vi "Get Cooler Status.vi"(8 "error in (no error)":errorcluster, 11 "CCDCamera in":refnum<class "CCDCamera.lvclass">) -> (0 "error out":errorcluster, 3 "CCDCamera out":refnum<class "CCDCamera.lvclass">)   [LabVIEW 2018, in "CCDCamera.lvclass"]
uses:
  CCDCamera.lvclass
  CCDCamera.lvclass/CCDCamera.ctl
  Cooler/Cooler.lvclass
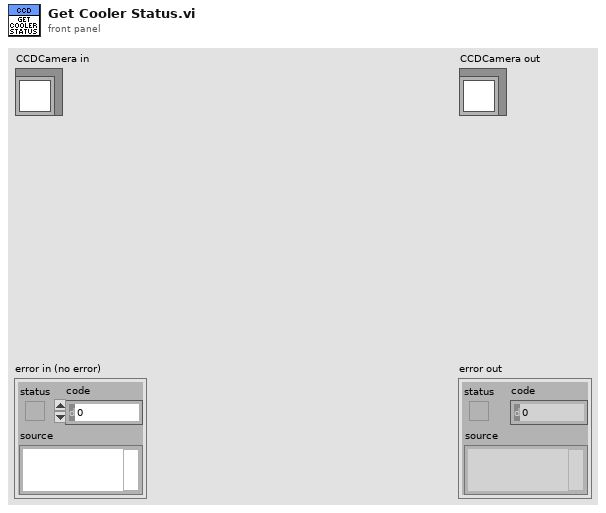
[diagram p1: front panel]
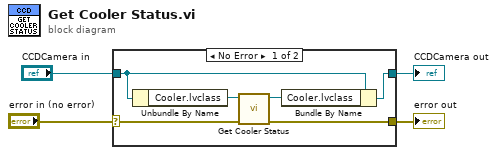
[diagram p0: block diagram]
diagram:
  n1 = case shown="No Error" "error in (no error)" {
    selector: "error in (no error)" -> [w5 w12]
    tunnel: [w6 w12] -> w3
    tunnel: [w8 w11] -> w1
    tunnel: "CCDCamera in" -> [w9 w11]
    frame No Error {
      n2 = Unbundle By Name(w9) -> ("Cooler.lvclass"=w10:refnum<class "Cooler.lvclass">)
      n3 = call "Get Cooler Status.vi"("error in (no error)"=w5, "Cooler in"=w10) -> ("error out"=w6:errorcluster, "Cooler out"=w7:refnum<class "Cooler.lvclass">)  [unwired: 8 in]
      n4 = Bundle By Name(cluster=w9, "Cooler.lvclass"=w7) -> (w8:refnum<class "CCDCamera.lvclass">)
    }
    frame Error {
    }
  }
  "error out" <- w3
  "CCDCamera out" <- w1
